vi "unzipEpub.vi"() -> ()   [LabVIEW 2016]
uses:
  <userlib>/_OpenG.lib/file/file.llb/Convert File Extension (Path)__ogtk.vi
  <userlib>/_OpenG.lib/array/array.llb/Sort 1D Array (I32)__ogtk.vi
  <userlib>/_OpenG.lib/array/array.llb/Index 1D Array Elements (Path)__ogtk.vi
panel:
  out "文件数":i32
  out "当前序号":i32
  out "PB":u32(slide) caption="完成" scale=0.0..1.0
  in  "确定按钮":bool
  in  "解压文件夹":path=path "D:/Downloads/Pic"
  in  "线程":i32=4
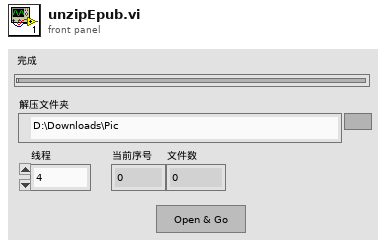
[diagram p1: front panel]
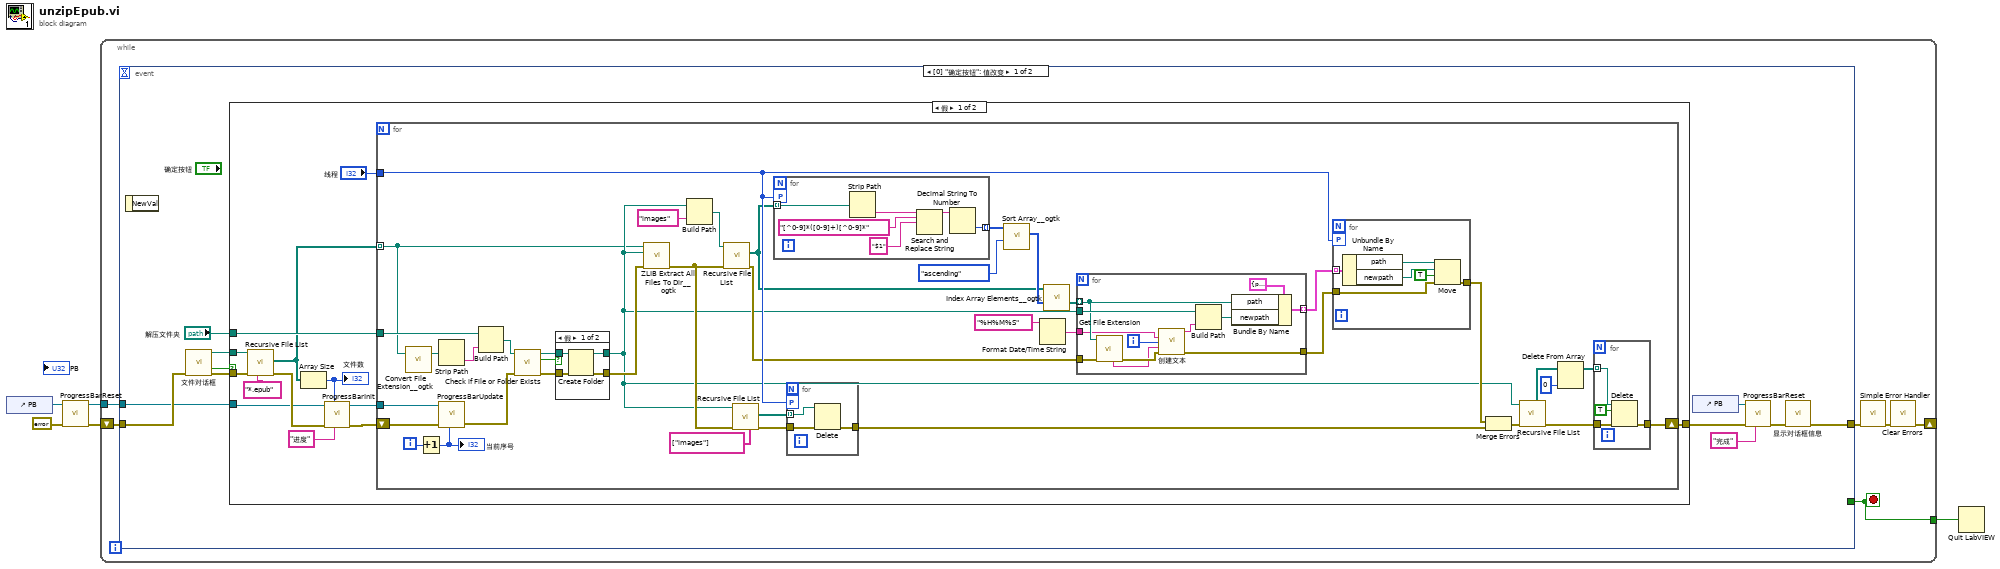
[diagram p0: block diagram]
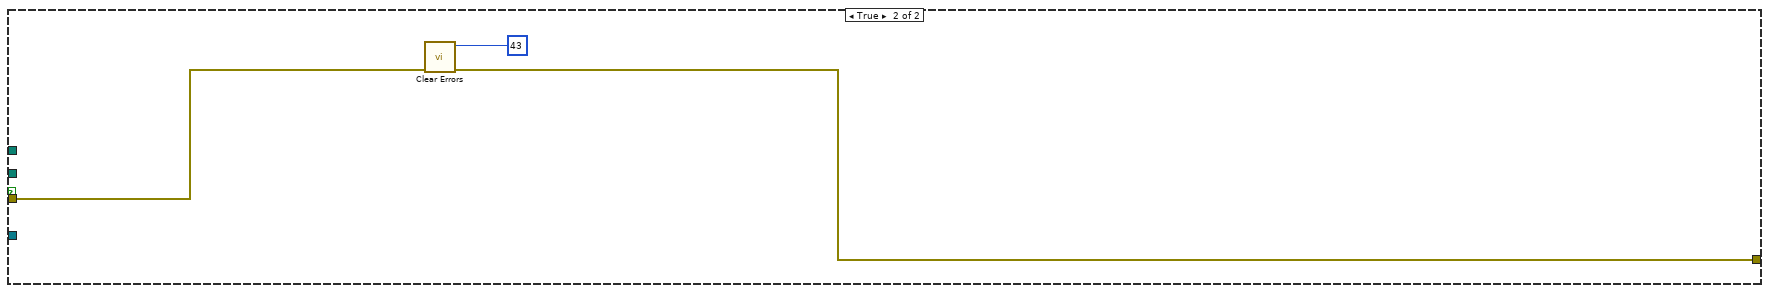
[diagram p3: hidden frame]
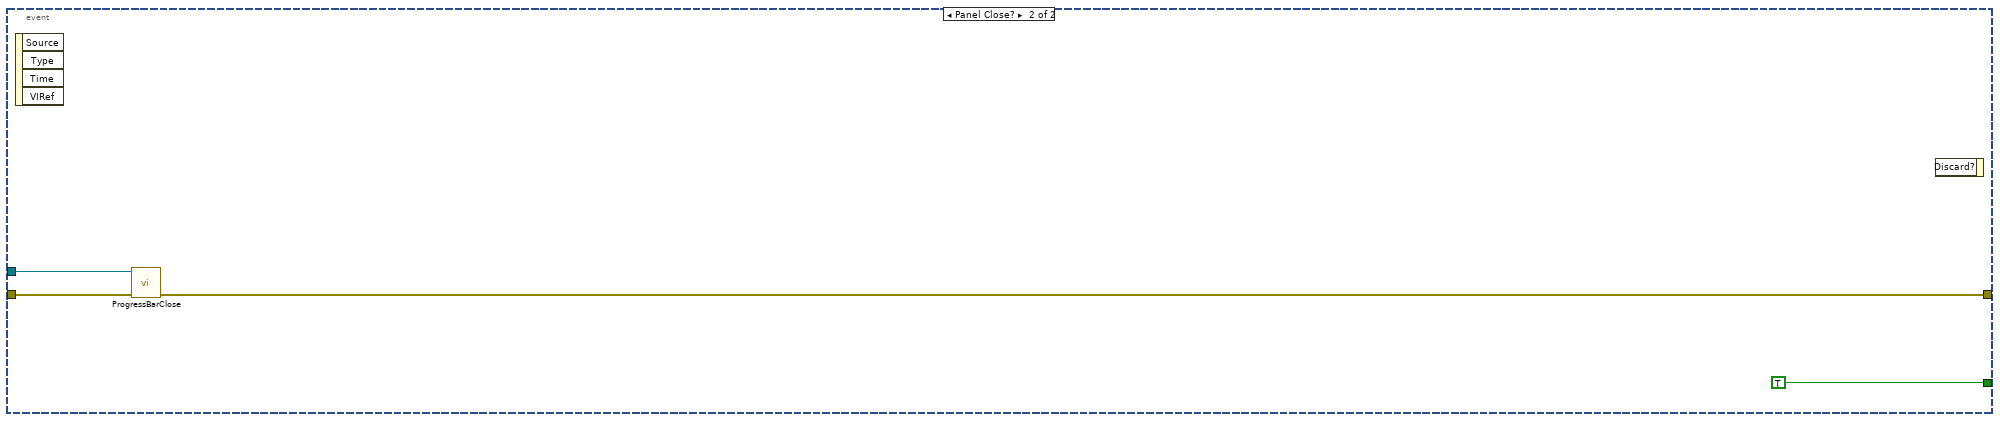
[diagram p4: hidden frame]
diagram:
  n1 = control-ref of="PB"() -> (w2:refnum<vi>)
  n2 = call <vilib>:"ProgressBarReset.vi"("Error in"=errorcluster {"status"=FALSE, "code"=0, "source"=""} ("error out"), "ProgressBar"=w2) -> ("Error out"=w3:errorcluster, "ProgressBarO"=w1:refnum<vi>)  [unwired: 8 in]
  n3 = while {
    shift-right: [w9] -> _
    shift-left: w3 -> [w8]
    tunnel: [w7] -> w4
    tunnel: w1 -> [w6]
    stop <- w7 stop-if-true
    n4 = event shown="[0] \"确定按钮\": 值改变" {
      selector: _ -> [_ _]
      dyn-events: _ -> [_ _]
      timeout: _ -> [_ _]
      tunnel: [w12 w117] -> w11
      tunnel: w8 -> [w17 w119]
      tunnel: [_ TRUE] -> w7
      tunnel: w6 -> [w16 w116]
      event "确定按钮": Value Change {
        n5 = event-data() -> ()  [unwired: 1 in, 1 out]
        n6 = call "文件对话框"("error in"=w17) -> ("selected path"=w20:path, "cancelled"=w22:bool, "error out"=w21:errorcluster)  [unwired: 11 in, 1 out]
        n7 = case shown="假" w22 {
          tunnel: w21 -> [w35 w115]
          tunnel: [w31 w114] -> w19
          tunnel: w20 -> [w33 _]
          tunnel: "解压文件夹" -> [w30 _]
          tunnel: w16 -> [w25 _]
          frame False {
            n8 = call <vilib>:"Recursive File List.vi"("pattern"="*.epub", "error in (no error)"=w35, "Folder Path"=w33) -> ("error out"=w34:errorcluster, "All Files in Dir"=w28:path[])  [unwired: 4 in, 3 out]
            n9 = Array Size(array=w28) -> (size(s)=w23:i32)
            "文件数" <- w23
            n10 = call <vilib>:"ProgressBarInit.vi"("Title"="进度", "Maximum"=w23, "Error in"=w34, "ProgressBar"=w25) -> ("Error out"=w29:errorcluster, "ProgressBarO"=w26:refnum<vi>)  [unwired: 6 in]
            n11 = for {
              tunnel: "线程" -> [w68]
              tunnel: w30 -> [w74]
              tunnel: w26 -> [w72]
              shift-right: [w75] -> w31
              shift-left: w29 -> [w70]
              tunnel: w28 -> [w36] mode=indexing
              i -> [w73]
              n12 = call-poly <userlib>:"Convert File Extension__ogtk.vi"("file name"=w36) -> ("new filename"=w50:path)  [unwired: 1 in, 1 out]
              n13 = Increment(x=w73) -> (x+1=w69:i32)
              "当前序号" <- w69
              n14 = Strip Path(path=w50) -> (name=w38:string)  [unwired: 1 out]
              n15 = call <vilib>:"ProgressBarUpdate.vi"("Value"=w69, "Error in"=w70, "ProgressBar"=w72) -> ("Error out"=w71:errorcluster)  [unwired: 7 in, 1 out]
              n16 = Build Path(base path=w74, name or relative path=w38) -> (appended path=w37:path)
              n17 = call <vilib>:"Check if File or Folder Exists.vi"("error in (no error)"=w71, "path"=w37) -> ("error out"=w54:errorcluster, "file or folder exists?"=w51:bool, "dup path"=w52:path)  [unwired: 7 in]
              n18 = case shown="假" w51 {
                tunnel: w54 -> [w86 w87]
                tunnel: [w85 w87] -> w53
                tunnel: w52 -> [w84 w88]
                tunnel: [w83 w88] -> w42
                frame False {
                  n19 = Create Folder(path (use dialog)=w84, error in=w86) -> (created path=w83:path, error out=w85:errorcluster)  [unwired: 1 in, 1 out]
                }
                frame True {
                }
              }
              n20 = call <userlib>:"ZLIB Extract All Files To Dir__ogtk.vi"("error in (no error)"=w53, "root directory (archive name without ending)"=w42, "archive name (file dialog)"=w36) -> ("error out"=w49:errorcluster)  [unwired: 6 in, 2 out]
              n21 = Build Path(base path=w42, name or relative path="images" ("名称或相对路径")) -> (appended path=w61:path)
              n22 = call <vilib>:"Recursive File List.vi"("error in (no error)"=w49, "Folder Path"=w61) -> ("error out"=w57:errorcluster, "All Files in Dir"=w63:path[])  [unwired: 5 in, 3 out]
              n23 = call <vilib>:"Recursive File List.vi"("Folders to Exclude"=string[] ["images"], "error in (no error)"=w49, "Folder Path"=w42) -> ("error out"=w47:errorcluster, "All Files in Dir"=w46:path[])  [unwired: 4 in, 3 out]
              n24 = for {
                tunnel: w63 -> [w112] mode=indexing
                tunnel: [w107] -> w66 mode=indexing
                workers-P: w68 -> [_]
                n25 = Strip Path(path=w112) -> (name=w111:string)  [unwired: 1 out]
                n26 = Search and Replace String(input string=w111, search string="[^0-9]*([0-9]+)[^0-9]*" ("搜索字符串"), replace string="$1" ("替换字符串(\"\")")) -> (result string=w108:string)  [unwired: 5 in, 3 out]
                n27 = Decimal String To Number(string=w108) -> (number=w107:i32)  [unwired: 2 in, 1 out]
              }
              n28 = for {
                tunnel: w47 -> [w82]
                tunnel: w46 -> [w81] mode=indexing
                tunnel: [w80] -> w44
                workers-P: w68 -> [_]
                n29 = Delete(path (use dialog)=w81, error in=w82) -> (error out=w80:errorcluster)  [unwired: 3 in, 2 out]
              }
              n30 = call-poly <userlib>:"Sort Array__ogtk.vi"("Order"=enum16{"ascending", "descending"}."ascending", "Array in"=w66) -> ("Sorted Pointers"=w64:i32[])  [unwired: 8 in, 1 out]
              n31 = Format Date/Time String(time format string (%c)="%H%M%S" ("时间格式字符串(%c)")) -> (date/time string=w59:string)  [unwired: 2 in]
              n32 = call-poly <userlib>:"Index Array Elements__ogtk.vi"("indices"=w64, "array"=w63) -> ("elements"=w62:path[])  [unwired: 9 in]
              n33 = for {
                tunnel: w62 -> [w97] mode=indexing
                tunnel: [w105] -> w58 mode=indexing
                tunnel: w42 -> [w98]
                tunnel: w59 -> [w95]
                tunnel: w57 -> [w101]
                tunnel: [w100] -> w56
                i -> [w104]
                n34 = call <vilib>:"Get File Extension.vi"("error in (no error)"=w101, "file"=w97) -> ("error out"=w99:errorcluster, "unmodified file extension"=w96:string)  [unwired: 5 in, 3 out]
                n35 = call "创建文本"("random"=w95, "idx"=w104, "extname"=w96, "error in (no error)"=w99) -> ("Result"=w103:string, "error out"=w100:errorcluster)  [unwired: 10 in]
                n36 = Build Path(base path=w98, name or relative path=w103) -> (appended path=w102:path)
                n37 = Bundle By Name(cluster=cluster{"newpath":path, "path":path} {"newpath"=path "", "path"=path ""} ("输出簇"), "path"=w97, "newpath"=w102) -> (w105:cluster{"newpath":path, "path":path})
              }
              n38 = for {
                tunnel: w58 -> [w94] mode=indexing
                workers-P: w68 -> [_]
                tunnel: w56 -> [w90]
                tunnel: [w89] -> w55
                n39 = Unbundle By Name(w94) -> ("path"=w93:path, "newpath"=w92:path)
                n40 = Move(source path=w93, error in=w90, 9:TRUE ("覆盖(F)"), 10:w92) -> (error out=w89:errorcluster)  [unwired: 1 in, 2 out]
              }
              n41 = Merge Errors(w55, w44) -> (w45:errorcluster)
              n42 = call <vilib>:"Recursive File List.vi"("error in (no error)"=w45, "Folder Path"=w42) -> ("error out"=w43:errorcluster, "All Folders"=w41:path[])  [unwired: 5 in, 3 out]
              n43 = Delete From Array(array=w41, index=0 ("索引")) -> (array with subset deleted=w39:path[])  [unwired: 1 in, 1 out]
              n44 = for {
                tunnel: w39 -> [w77] mode=indexing
                tunnel: w43 -> [w79]
                tunnel: [w78] -> w75
                n45 = Delete(path (use dialog)=w77, entire hierarchy (F)=TRUE ("整个层次结构(F)"), error in=w79) -> (error out=w78:errorcluster)  [unwired: 2 in, 2 out]
              }
            }
          }
          frame True {
            n46 = call <vilib>:"Clear Errors.vi"("error in (no error)"=w115, "specific error code to clear (0: all)"=43) -> ("error out"=w114:errorcluster)  [unwired: 4 in, 1 out]
          }
        }
        n47 = control-ref of="PB"() -> (w13:refnum<vi>)
        n48 = call <vilib>:"ProgressBarReset.vi"("Title"="完成", "Error in"=w19, "ProgressBar"=w13) -> ("Error out"=w15:errorcluster)  [unwired: 7 in, 1 out]
        n49 = call "显示对话框信息"("error in (no error)"=w15) -> ("error out"=w12:errorcluster)  [unwired: 9 in, 1 out]
      }
      event Panel Close? {
        n50 = event-data() -> ()  [unwired: 1 in, 4 out]
        n51 = call <vilib>:"ProgressBarClose.vi"("Error in"=w119, "ProgressBar"=w116) -> ("Error out"=w117:errorcluster)  [unwired: 9 in]
        n52 = event-data() -> ()  [unwired: 2 in, 1 out]
      }
    }
    n53 = call <vilib>:"Simple Error Handler.vi"("error in (no error)"=w11) -> ("error out"=w10:errorcluster)  [unwired: 4 in, 4 out]
    n54 = call <vilib>:"Clear Errors.vi"("error in (no error)"=w10) -> ("error out"=w9:errorcluster)  [unwired: 5 in, 1 out]
  }
  n55 = Quit LabVIEW(quit? (T)=w4) -> ()
